vi "App Settings.vi"(8 "Error in (no error)":errorcluster) -> (0 "Error out":errorcluster)   [LabVIEW 2022 SP3]
uses:
  Controls/Settings States.ctl
  Controls/Application Settings.ctl
  <userlib>/_MGI/Error Reporter/MGI Error Reporter Base/MGI Error Reporter Base.lvclass
panel:
  in  "Cancel":bool
  in  "Save Settings":bool
  in  "Settings Tab":T1(tab)
  in  "Component Name Prefix":string
  in  "Enable Secondary":bool caption="Enable"
  in  "Backup Storage Location":path
  in  "Enable Primary":bool caption="Enable"
  in  "Primary Storage Location":path
  in  "Image Averaging Option":bool
  # "Application Settings"
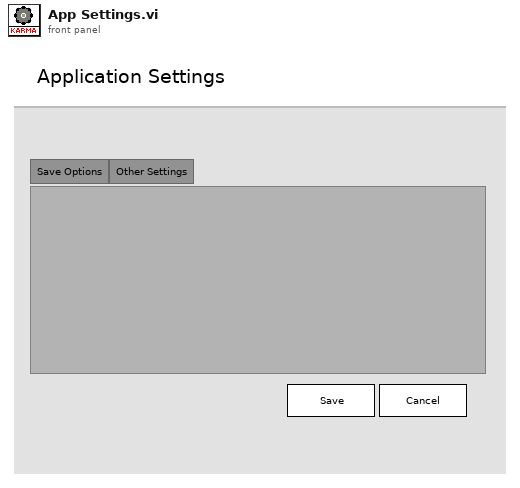
[diagram p1: front panel]
types:
  T1 = enum32{"Sensor Settings", "Save Options", "Other Settings"}
  T2 = typedef "Settings States.ctl" = enum16{"Poll UI", "Initialize", "Save", "Exit", "Error"}
  T3 = typedef "Application Settings.ctl" = cluster{"Save Options":cluster{"Primary Storage Location":path, "Backup Storage Location":path, "Enable Primary":bool, "Enable Secondary":bool}, "Other Settings":cluster{"Show Image Averaging Option":bool, "Component Name Prefix":string}}
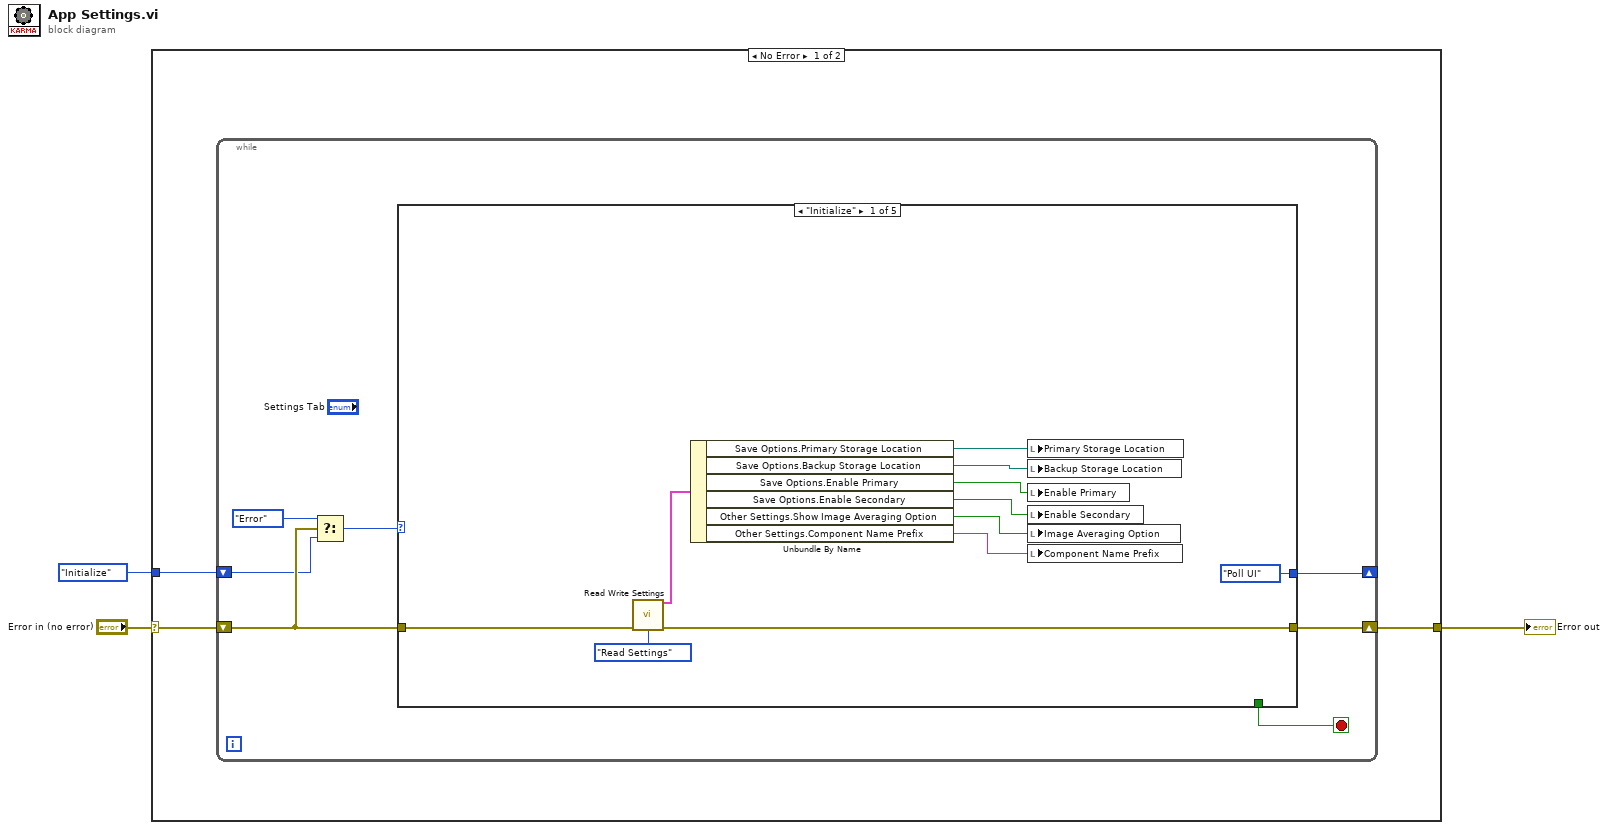
[diagram p0: block diagram]
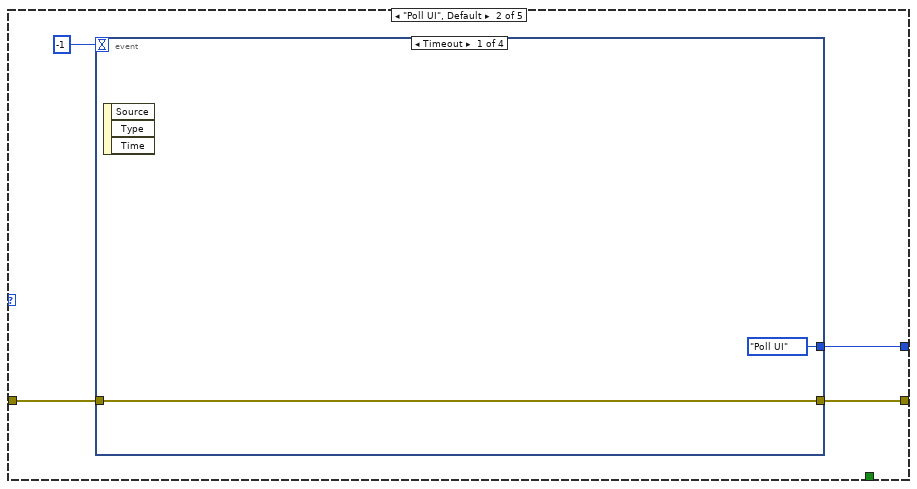
[diagram p2: hidden frame]
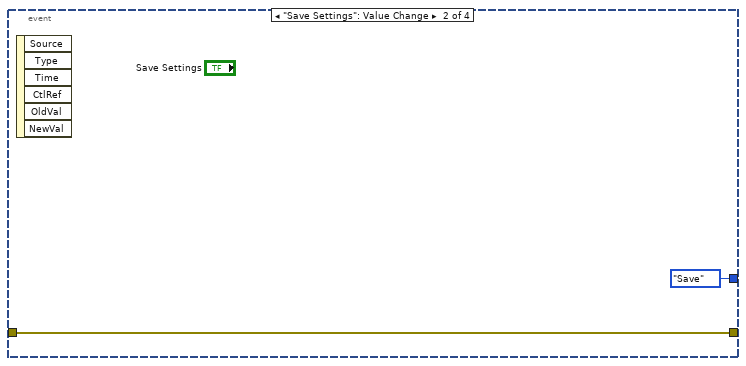
[diagram p3: hidden frame]
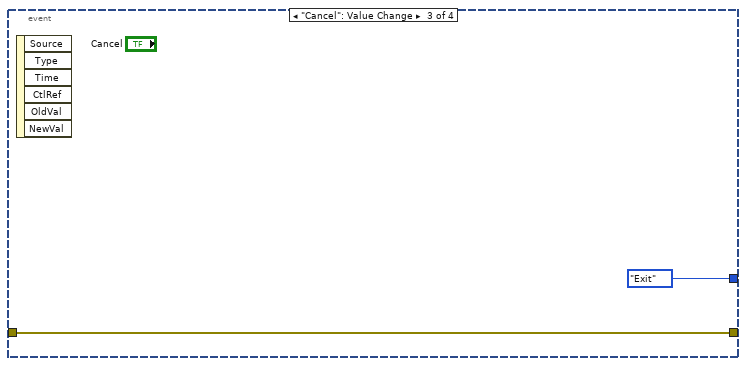
[diagram p4: hidden frame]
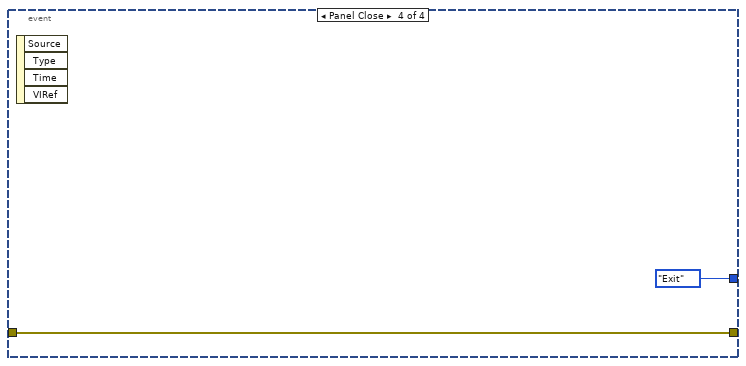
[diagram p5: hidden frame]
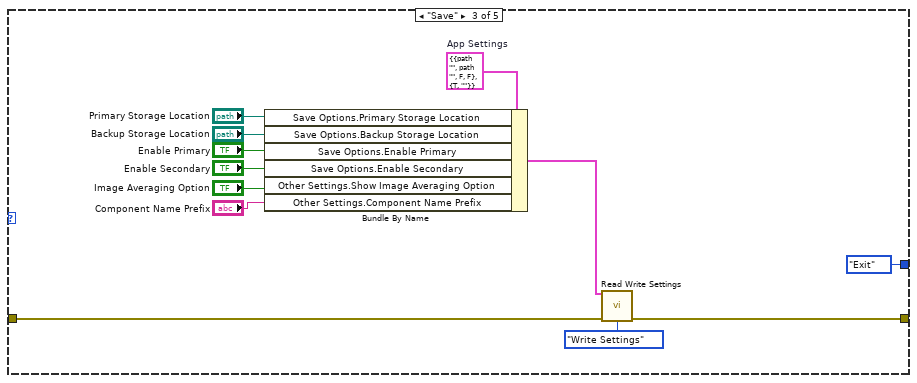
[diagram p6: hidden frame]
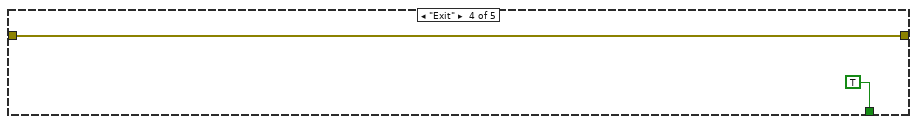
[diagram p7: hidden frame]
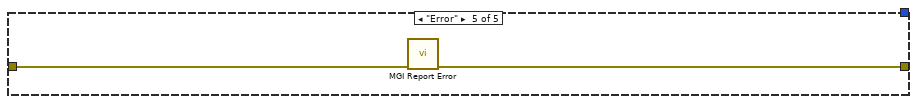
[diagram p8: hidden frame]
diagram:
  n1 = case shown="No Error" "Error in (no error)" {
    selector: "Error in (no error)" -> [w4 w53]
    tunnel: Settings_States."Initialize" -> [w6 _]
    tunnel: [w5 w53] -> w2
    frame No Error {
      n2 = while {
        shift-right: [w8] -> _
        shift-left: w6 -> [w11]
        shift-right: [w9] -> w5
        shift-left: w4 -> [w13]
        stop <- w7 stop-if-true
        n3 = Select(t=Settings_States."Error", s=w13, f=w11) -> (s? t:f=w10:T2)
        n4 = case shown="\"Initialize\"" w10 {
          tunnel: w13 -> [w23 w28 w45 w50 w52]
          tunnel: [w22 w27 w44 w50 w51] -> w9
          tunnel: [Settings_States."Poll UI" w25 Settings_States."Exit" _ _] -> w8
          tunnel: [_ _ _ TRUE _] -> w7
          frame "Initialize" {
            n5 = call "Read Write Settings.vi"("error in (no error)"=w23, "Operations"=enum16{"Read Settings", "Write Settings"}."Read Settings") -> ("Settings Out"=w20:T3, "error out"=w22:errorcluster)  [unwired: 12 in]
            n6 = Unbundle By Name(w20) -> ("Save Options.Primary Storage Location"=w19:path, "Save Options.Backup Storage Location"=w18:path, "Save Options.Enable Primary"=w17:bool, "Save Options.Enable Secondary"=w16:bool, "Other Settings.Show Image Averaging Option"=w15:bool, "Other Settings.Component Name Prefix"=w14:string)
            n7 = local write "Primary Storage Location"(w19) -> ()
            n8 = local write "Backup Storage Location"(w18) -> ()
            n9 = local write "Enable Primary"(w17) -> ()
            n10 = local write "Enable Secondary"(w16) -> ()
            n11 = local write "Image Averaging Option"(w15) -> ()
            n12 = local write "Component Name Prefix"(w14) -> ()
          }
          frame "Poll UI", Default {
            n13 = event shown="[0] Timeout" {
              selector: _ -> [_ _ _ _]
              dyn-events: _ -> [_ _ _ _]
              timeout: -1 -> [_ _ _ _]
              tunnel: w28 -> [w30 w32 w34 w36]
              tunnel: [w30 w32 w34 w36] -> w27
              tunnel: [Settings_States."Poll UI" Settings_States."Save" Settings_States."Exit" Settings_States."Exit"] -> w25
              event Timeout {
                n14 = event-data() -> ()  [unwired: 1 in, 3 out]
              }
              event "Save Settings": Value Change {
                n15 = event-data() -> ()  [unwired: 1 in, 6 out]
              }
              event "Cancel": Value Change {
                n16 = event-data() -> ()  [unwired: 1 in, 6 out]
              }
              event Panel Close {
                n17 = event-data() -> ()  [unwired: 1 in, 4 out]
              }
            }
          }
          frame "Save" {
            w48 = T3 {"Save Options"={"Primary Storage Location"=path "", "Backup Storage Location"=path "", "Enable Primary"=FALSE, "Enable Secondary"=FALSE}, "Other Settings"={"Show Image Averaging Option"=TRUE, "Component Name Prefix"=""}}  # App Settings
            n18 = Bundle By Name(cluster=w48, "Save Options.Primary Storage Location"="Primary Storage Location", "Save Options.Backup Storage Location"="Backup Storage Location", "Save Options.Enable Primary"="Enable Primary", "Save Options.Enable Secondary"="Enable Secondary", "Other Settings.Show Image Averaging Option"="Image Averaging Option", "Other Settings.Component Name Prefix"="Component Name Prefix") -> (w42:T3)
            n19 = call "Read Write Settings.vi"("Settings In"=w42, "error in (no error)"=w45, "Operations"=enum16{"Read Settings", "Write Settings"}."Write Settings") -> ("error out"=w44:errorcluster)  [unwired: 11 in, 1 out]
          }
          frame "Exit" {
          }
          frame "Error" {
            n20 = call <userlib>:"MGI Report Error.vi"("error in"=w52) -> ("no error"=w51:errorcluster)  [unwired: 10 in]
          }
        }
      }
    }
    frame Error {
    }
  }
  "Error out" <- w2
